vi "niRFSysCalReader Cal Path Info Variant Name.vi"() -> (3 "Cal Path Info Name":string)   [LabVIEW 2016, in "niRFSysCalReader.lvlib"]
uses:
  niRFSysCalReader.lvlib
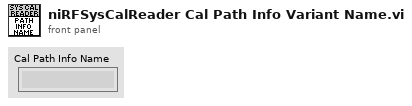
[diagram p1: front panel]
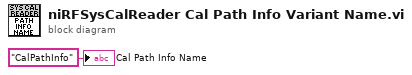
[diagram p0: block diagram]
diagram:
  "Cal Path Info Name" <- "CalPathInfo" ("name")
